vi "Time.vi"(8 "error in (no error)":errorcluster, 10 "Control In":T1, 11 "C4 Dispense in":refnum<class "Iterative Dispense.lvclass">) -> (0 "error out":errorcluster, 1 "Timing Data":i32[](array[numeric]), 2 "Control Out":T1, 3 "C4 Dispense out":refnum<class "Iterative Dispense.lvclass">)   [LabVIEW 2020, in "Iterative Dispense.lvclass"]
uses:
  Iterative Dispense.lvclass
  Controller/Controllers.ctl
  Controller/I-O/I-O.lvclass
  Controller/Dispenser/Dispenser.lvclass
  C:/Program Files (x86)/Aerotech/A3200/LabVIEW/2010/Bin/Aerotech.A3200.dll
  Program Files (x86)/Aerotech/A3200/LabVIEW/2010/Bin/Aerotech.A3200.dll
  Iterative Dispense.lvclass/Iterative Dispense.ctl
  Controller/Motion/Motion.lvclass
  Controller/Motion/A3200/A3200.lvclass
  Controller/Controller.lvclass
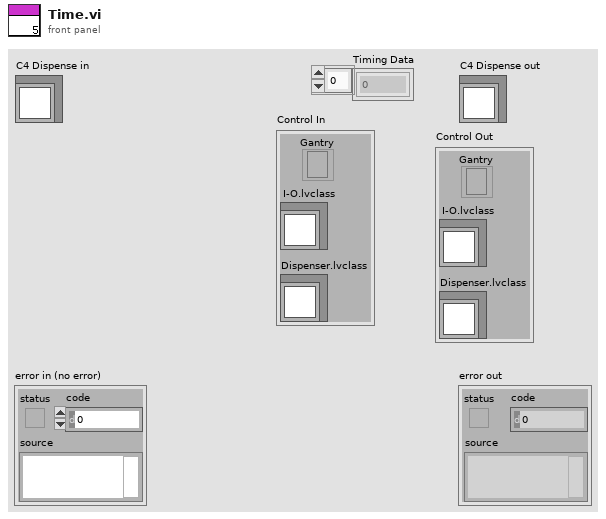
[diagram p1: front panel]
types:
  T1 = typedef "Controller.lvclass/Controllers.ctl" = cluster{"I-O.lvclass":refnum<class "I-O.lvclass">, "Dispenser.lvclass":refnum<class "Dispenser.lvclass">, "Gantry":refnum<k24>}
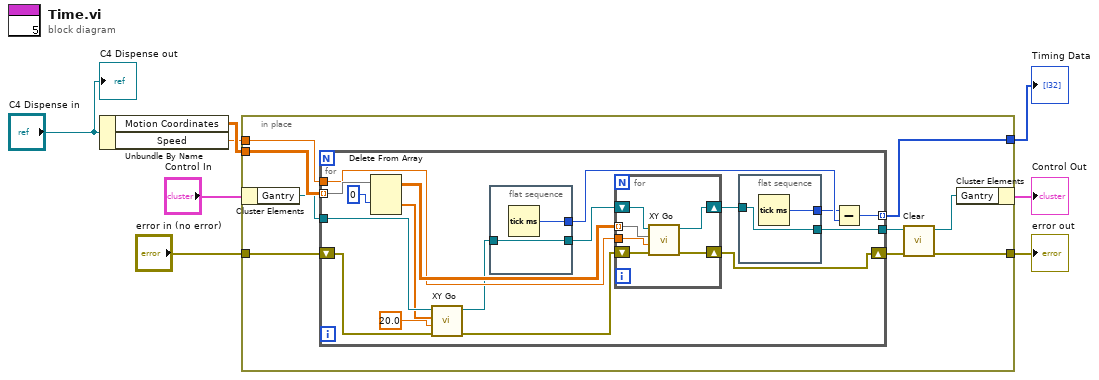
[diagram p0: block diagram]
diagram:
  n1 = Unbundle By Name("C4 Dispense in") -> ("Motion Coordinates"=w8:dbl[][][], "Speed"=w3:dbl)
  n2 = in-place {
    in-place-border: w8 -> [w17]
    in-place-border: [w16] -> w7
    in-place-border: w3 -> [w15]
    in-place-border: "error in (no error)" -> [w11]
    in-place-border: [w9] -> w1
    n3 = in-place-cluster #1("Control In") -> ("Gantry"=w14:refnum<k24>)
    n4 = for {
      tunnel: [w32] -> w16 mode=indexing
      tunnel: w17 -> [w29] mode=indexing
      tunnel: w15 -> [w28]
      tunnel: w14 -> [w26]
      tunnel: [w23] -> w12
      shift-right: [w18] -> w10
      shift-left: w11 -> [w20]
      n5 = Delete From Array(array=w29, index (row)=0) -> (deleted portion=w22:dbl[], array with subset deleted=w31:dbl[][])  [unwired: 2 in]
      n6 = call "XY Go.vi"("error in (no error)"=w20, "Speed"=20.0, "XY"=w22, "Gantry 2"=w26) -> ("error out"=w19:errorcluster, "Gantry 3"=w25:refnum<k24>)  [unwired: 6 in]
      n7 = flat-sequence {
        tunnel: [w38] -> w34
        tunnel: w25 -> [w37]
        tunnel: [w37] -> w24
        frame #0 {
          n8 = Tick Count (ms)() -> (millisecond timer value=w38:u32)
        }
      }
      n9 = for {
        tunnel: w31 -> [w42] mode=indexing
        tunnel: w28 -> [w41]
        shift-right: [w43] -> w27
        shift-left: w24 -> [w44]
        shift-right: [w39] -> w18
        shift-left: w19 -> [w40]
        n10 = call "XY Go.vi"("error in (no error)"=w40, "Speed"=w41, "XY"=w42, "Gantry 2"=w44) -> ("error out"=w39:errorcluster, "Gantry 3"=w43:refnum<k24>)  [unwired: 6 in]
      }
      n11 = flat-sequence {
        tunnel: [w36] -> w33
        tunnel: [w35] -> w23
        tunnel: w27 -> [w35]
        frame #0 {
          n12 = Tick Count (ms)() -> (millisecond timer value=w36:u32)
        }
      }
      n13 = Subtract(x=w33, y=w34) -> (x-y=w32:u32)
    }
    n14 = call "Clear.vi"("error in (no error)"=w10, "Gantry 2"=w12) -> ("error out"=w9:errorcluster, "Gantry 3"=w13:refnum<k24>)  [unwired: 8 in]
    n15 = in-place-cluster #1("Gantry"=w13) -> (→"Control Out":T1)
  }
  "error out" <- w1
  "Timing Data" <- w7
  "C4 Dispense out" <- "C4 Dispense in"
